vi "VoltScale.vi"(5 "instrument handle in":refnum<k15>, 6 "Channel name":string, 7 "error in":errorcluster) -> (0 "inst handle OUT":refnum<k15>, 1 "V/ div":string, 2 "FS Volt pp":dbl format="%.2f", 3 "error out":errorcluster)   [LabVIEW 2022 SP3]
panel:
  out "Att dB":dbl format="%.2f"
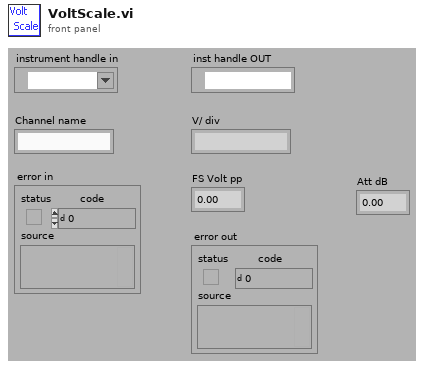
[diagram p1: front panel]
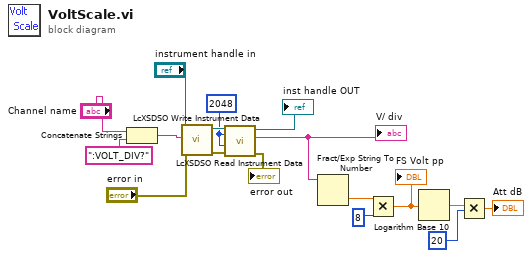
[diagram p0: block diagram]
diagram:
  w1 = 2048
  n1 = Concatenate Strings("Channel name", ":VOLT_DIV?") -> (w8:string)
  n2 = call "LcXSDSO Write Instrument Data.vi"("error in (no error)"="error in", "write buffer"=w8, "instrument handle"="instrument handle in") -> ("error out"=w5:errorcluster, "instrument handle out"=w4:refnum<k15>)  [unwired: 7 in]
  n3 = call "LcXSDSO Read Instrument Data.vi"("error in (no error)"=w5, "size of read buffer"=w1, "number of bytes to read"=w1, "instrument handle"=w4) -> ("error out"=→"error out":errorcluster, "read buffer"=w11:string, "instrument handle out"=→"inst handle OUT":refnum<k15>)  [unwired: 4 in, 1 out]
  "V/ div" <- w11
  n4 = Fract/Exp String To Number(string=w11) -> (number=w12:dbl)  [unwired: 3 in, 1 out]
  n5 = Multiply(x=w12, y=8) -> (x*y=w17:dbl)
  "FS Volt pp" <- w17
  n6 = Logarithm Base 10(1:w17) -> (0:w14:dbl)
  n7 = Multiply(x=w14, y=20) -> (x*y=→"Att dB":dbl)
